vi "Quad Range.vi"(1 "Transmission Quad B read":dbl, 2 "Transmission Quad A set":dbl, 3 "Transmission Quad A read":dbl, 4 "Transmission Quad B set":dbl) -> (0 "Quad range?":bool)   [LabVIEW 2016, in "Transmission.lvlib"]
doc: "This takes the quad ranges and combines them into one output boolean"
uses:
  Transmission.lvlib
  Low Energy End/Low energy.lvlib
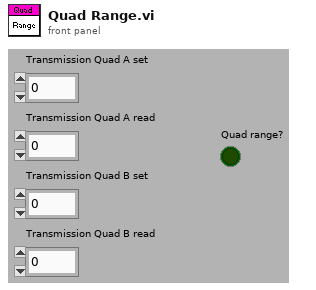
[diagram p1: front panel]
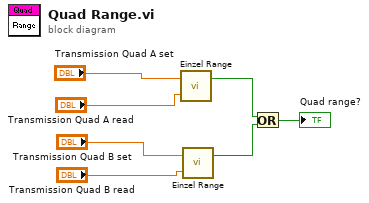
[diagram p0: block diagram]
diagram:
  n1 = call "Einzel Range.vi"("Inj image Readback"="Transmission Quad A read", "Inj image Einzel Set"="Transmission Quad A set") -> ("Einzel  Range"=w2:bool)  [unwired: 1 out]
  n2 = call "Einzel Range.vi"("Inj image Readback"="Transmission Quad B read", "Inj image Einzel Set"="Transmission Quad B set") -> ("Einzel  Range"=w3:bool)  [unwired: 1 out]
  n3 = Or(x=w2, y=w3) -> (x .or. y?=→"Quad range?":bool)
